vi "SLICER_TESTER.vi"() -> ()   [LabVIEW 2016]
panel:
  out "Intensity info plot":dbl[][](graph)
  out "Intensity Graph":dbl[][](graph)
  out "Intensity Info OUT":cluster{dbl[], dbl[]}[](array[cluster])
  out "error out":errorcluster
  in  "error in (no error)":errorcluster
  in  "X":T1(ring)
  in  "X AXIS":i32(listbox)
  in  "Z":T1(ring)
  in  "Y AXIS":i32(listbox)
  in  "Fast":dbl(slide) scale=0.0..44.0
  in  "Slowest":dbl(slide) scale=0.0..10.0
  in  "Slow":dbl(slide) scale=0.0..10.0
  in  "Big Ol Array IN":T2(array[cluster])
  in  "stop":bool
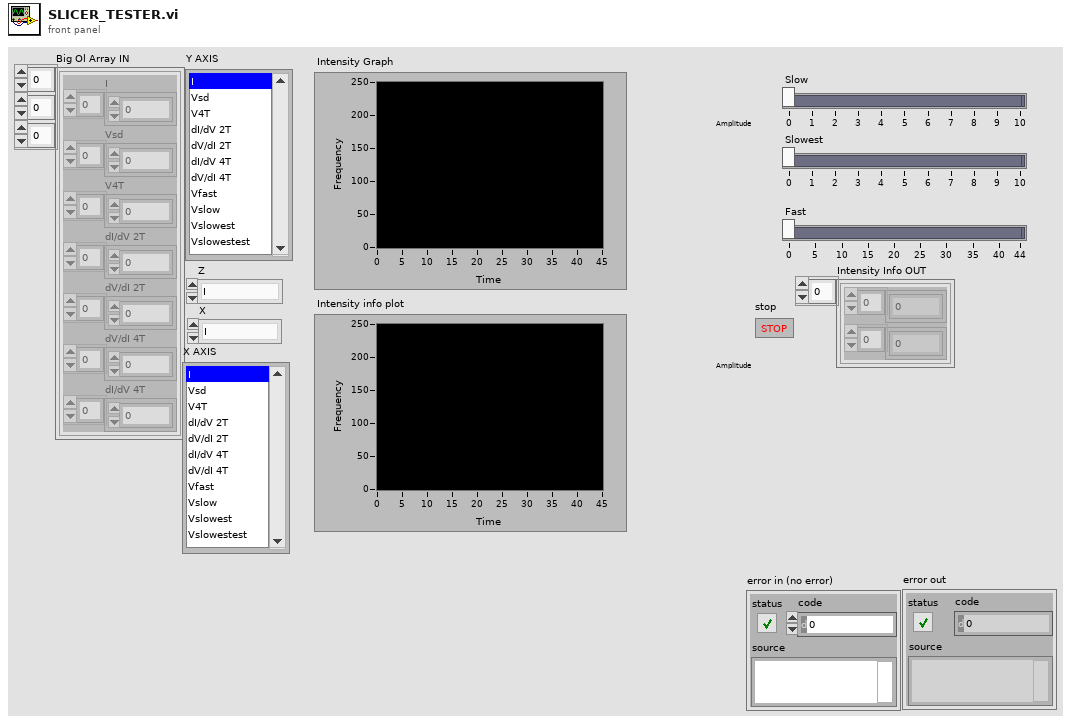
[diagram p1: front panel]
types:
  T1 = enum16{"I", "Vsd", "V4T", "dI/dV 2T", "dV/dI 2T", "dV/dI 4T", "dI/dV 4T"}
  T2 = cluster{"I":dbl[], "Vsd":dbl[], "V4T":dbl[], "dI/dV 2T":dbl[], "dV/dI 2T":dbl[], "dV/dI 4T":dbl[], "dI/dV 4T":dbl[]}[][][]
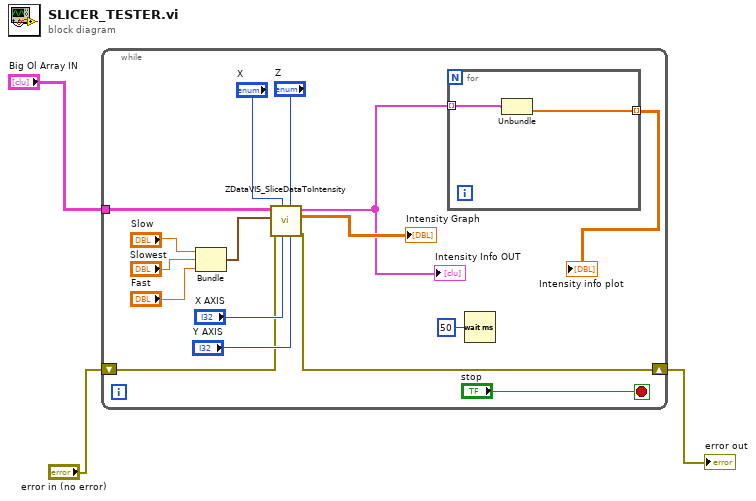
[diagram p0: block diagram]
diagram:
  n1 = while {
    tunnel: "Big Ol Array IN" -> [w17]
    shift-right: [w8] -> w1
    shift-left: "error in (no error)" -> [w7]
    stop <- "stop" stop-if-true
    n2 = Bundle("Slow"="Slow", "Slowest"="Slowest", "Fast"="Fast") -> (w13:cluster{"Slow":dbl, "Slowest":dbl, "Fast":dbl})  [unwired: 1 in]
    n3 = call "ZDataVIS_SliceDataToIntensity.vi"("Y AXIS"="Y AXIS", "Z"="Z", "X AXIS"="X AXIS", "X"="X", "error in (no error)"=w7, "Outer Indices"=w13, "Big Ol Array IN"=w17) -> ("error out"=w8:errorcluster, "Intensity Graph"=→"Intensity Graph":dbl[][], "Intensity Info OUT"=w5:cluster{dbl[], dbl[]}[])  [unwired: 2 in]
    "Intensity Info OUT" <- w5
    n4 = for {
      tunnel: w5 -> [w21] mode=indexing
      tunnel: [w20] -> w4 mode=indexing
      n5 = Unbundle(w21) -> (w20:dbl[])  [unwired: 1 out]
    }
    "Intensity info plot" <- w4
    n6 = Wait (ms)(milliseconds to wait=u32 50) -> ()  [unwired: 1 out]
  }
  "error out" <- w1
